vi "Init Formatter Runtime.vi"(8 "error in (no error)":errorcluster, 11 "Report Config in":refnum<class "Report Config.lvclass">) -> (0 "error out":errorcluster, 2 "Formatters":refnum<class "Formatter.lvclass">[](array[class]), 3 "Report Config out":refnum<class "Report Config.lvclass">)   [LabVIEW 2015, in "Report Config.lvclass"]
doc: "This VI calls the init runtime for all configured formatters and returns the runtime class for those formatters."
uses:
  Report Config.lvclass
  Report Formatters/Base Class/Config/Formatter Config.lvclass
  Report Formatters/Base Class/Execution/Formatter.lvclass
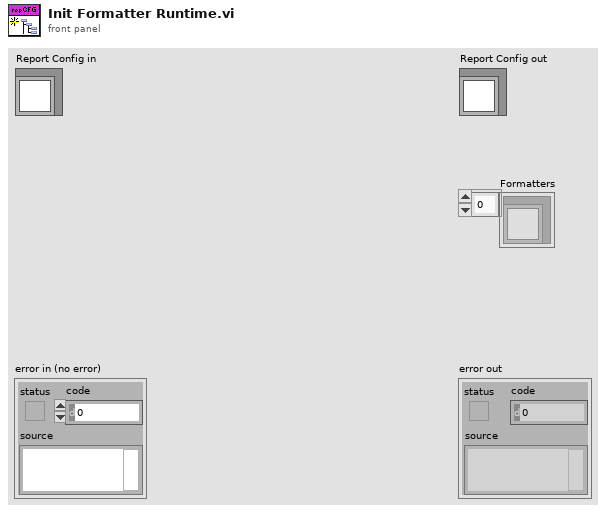
[diagram p1: front panel]
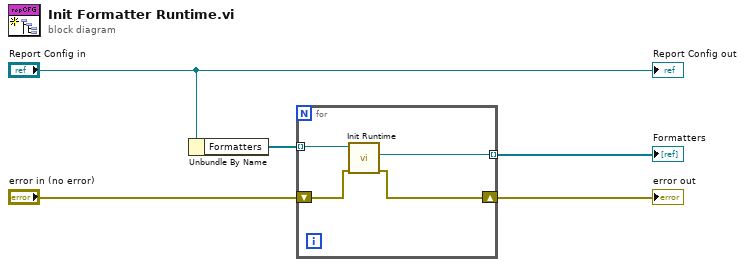
[diagram p0: block diagram]
diagram:
  n1 = Unbundle By Name("Report Config in") -> ("Formatters"=w1:refnum<class "Formatter Config.lvclass">[])
  n2 = for {
    tunnel: w1 -> [w9] mode=indexing
    tunnel: [w8] -> w2 mode=indexing
    shift-right: [w6] -> w4
    shift-left: "error in (no error)" -> [w7]
    n3 = call-dynamic "Init Runtime.vi"("error in (no error)"=w7, "Formatter Config in"=w9) -> ("error out"=w6:errorcluster, "Formatter.lvclass"=w8:refnum<class "Formatter.lvclass">)  [unwired: 7 in, 1 out]
  }
  "error out" <- w4
  "Formatters" <- w2
  "Report Config out" <- "Report Config in"
